vi "test Echo Frame.vi"(11 "Test Case In":refnum<class "Test PCANBasic.lvclass">) -> (0 "error out":errorcluster, 3 "Test Case Out":refnum<class "Test PCANBasic.lvclass">)   [LabVIEW 2020, in "Test PCANBasic.lvclass"]
uses:
  Test PCANBasic.lvclass
  C:/Program Files/National Instruments/LabVIEW 2026/vi.lib/Astemes/LUnit/Test Case.lvclass
  <vilib>/Astemes/LUnit/Test Case.lvclass/Test Case.ctl
  Test PCANBasic.lvclass/Test PCANBasic.ctl
  C:/Program Files/National Instruments/LabVIEW 2026/vi.lib/Astemes/LUnit/LUnit Runnable.lvclass
  D:/git/PCAN-Basic-LabVIEW/tests/Tests PCANBasic/Test PCANBasic.lvclass
  source/PCANBasic.lvlib
  Global PCAN Channel.vi
  Global PCAN Baudrate.vi
  <vilib>/Astemes/LUnit/Test Case.lvclass
panel:
  out "PCAN Message":T1 {"DATA"."7" format="%.0x"; "DATA"."6" format="%.0x"; "DATA"."5" format="%.0x"; "DATA"."4" format="%.0x"; "DATA"."3" format="%.0x"; "DATA"."2" format="%.0x"; "DATA"."1" format="%.0x"; "DATA"."0" format="%.0x"; "MSGTYPE"."Type" items=["STANDARD"=0, "RTR"=1, "ERRFRAME"=64, "STATUS"=128]}
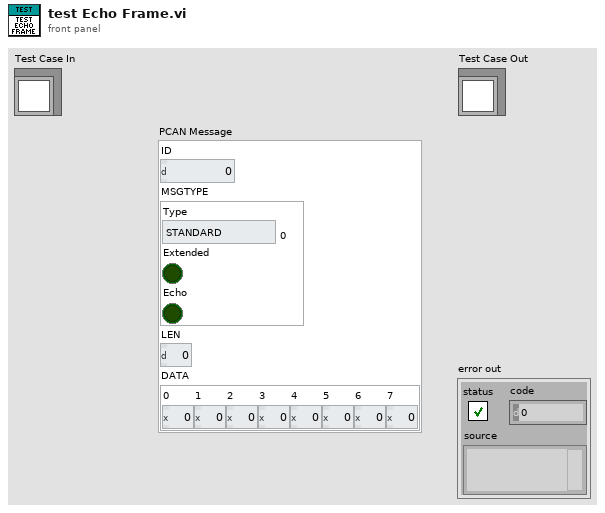
[diagram p1: front panel]
types:
  T1 = cluster{"ID":u32, "MSGTYPE":cluster{"Type":u8, "Extended":bool, "Echo":bool}, "LEN":u8, "DATA":cluster{"0":u8, "1":u8, "2":u8, "3":u8, "4":u8, "5":u8, "6":u8, "7":u8}}
  T2 = cluster{"0":u8, "1":u8, "2":u8, "3":u8, "4":u8, "5":u8, "6":u8, "7":u8}
  T3 = typedef "PCANBasic.lvlib/PCAN Baud.ctl" = u16
  T4 = typedef "PCANBasic.lvlib/TPCANHandle.ctl" = u16
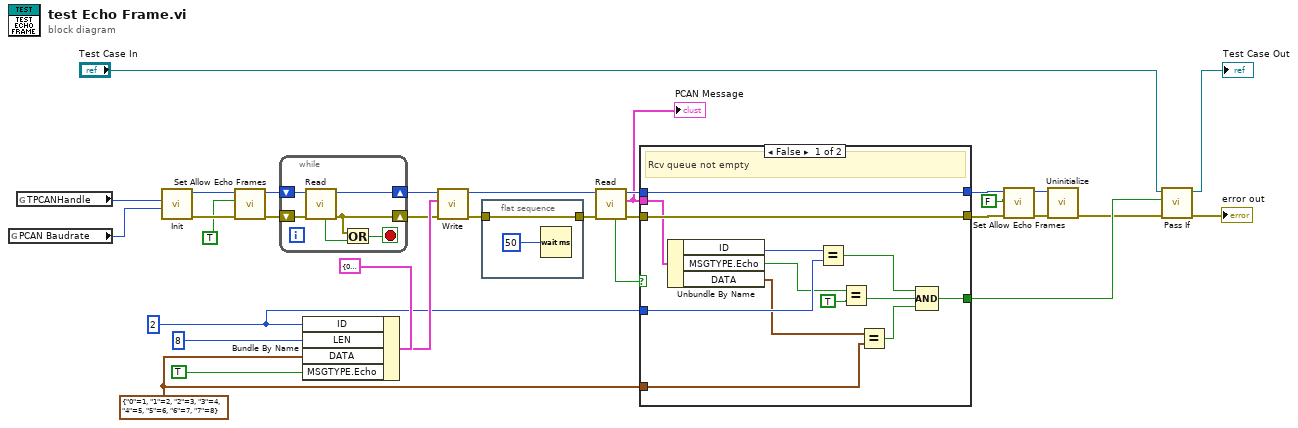
[diagram p0: block diagram]
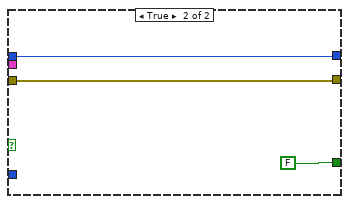
[diagram p2: hidden frame]
diagram:
  w16 = T2 {"0"=1, "1"=2, "2"=3, "3"=4, "4"=5, "5"=6, "6"=7, "7"=8} ("DATA")
  w17 = u32 2 ("ID")
  n1 = global read "Global PCAN Baudrate.vi" "PCAN Baudrate"() -> (w29:T3)
  n2 = global read "Global PCAN Channel.vi" "TPCANHandle"() -> (w28:T4)
  n3 = call "Init.vi"("Baudrate"=w29, "Channel"=w28) -> ("error out"=w27:errorcluster, "TPCANHandle out"=w12:T4)  [unwired: 7 in, 1 out]
  n4 = call "Set Allow Echo Frames.vi"("error in"=w27, "Enable"=TRUE, "TPCANHandle in"=w12) -> ("error out"=w13:errorcluster, "TPCANHandle out"=w10:T4)  [unwired: 6 in, 1 out]
  n5 = while {
    shift-right: [w34] -> w22
    shift-left: w13 -> [w38]
    shift-right: [w36] -> w21
    shift-left: w10 -> [w37]
    stop <- w33 stop-if-true
    n6 = call "Read.vi"("error in"=w38, "TPCANHandle in"=w37) -> ("error out"=w34:errorcluster, "TPCANHandle out"=w36:T4, "Receive Queue empty"=w35:bool)  [unwired: 4 in, 3 out]
    n7 = Or(x=w34, y=w35) -> (x .or. y?=w33:bool)
  }
  n8 = Bundle By Name(cluster=T1 {"ID"=0, "MSGTYPE"={"Type"=0, "Extended"=FALSE, "Echo"=FALSE}, "LEN"=0, "DATA"={"0"=0, "1"=0, "2"=0, "3"=0, "4"=0, "5"=0, "6"=0, "7"=0}} ("PCAN Message"), "ID"=w17, "LEN"=u8 8, "DATA"=w16, "MSGTYPE.Echo"=TRUE) -> (w24:T1)
  n9 = call "Write.vi"("error in"=w22, "PCAN Message"=w24, "TPCANHandle in"=w21) -> ("error out"=w7:errorcluster, "TPCANHandle out"=w19:T4)  [unwired: 6 in, 1 out]
  n10 = flat-sequence {
    tunnel: w7 -> [w40]
    tunnel: [w40] -> w6
    frame #0 {
      n11 = Wait (ms)(milliseconds to wait=u32 50) -> ()  [unwired: 1 out]
    }
  }
  n12 = call "Read.vi"("error in"=w6, "TPCANHandle in"=w19) -> ("error out"=w20:errorcluster, "PCAN Message"=w5:T1, "TPCANHandle out"=w18:T4, "Receive Queue empty"=w14:bool)  [unwired: 4 in, 2 out]
  "PCAN Message" <- w5
  n13 = case shown="False" w14 {
    tunnel: w20 -> [w43 w55]
    tunnel: w18 -> [w42 w54]
    tunnel: [w43 w55] -> w9
    tunnel: w5 -> [w41 _]
    tunnel: w17 -> [w53 _]
    tunnel: w16 -> [w48 _]
    tunnel: [w44 FALSE] -> w15
    tunnel: [w42 w54] -> w3
    frame False {
      # "Rcv queue not empty"
      n14 = Unbundle By Name(w41) -> ("ID"=w52:u32, "MSGTYPE.Echo"=w51:bool, "DATA"=w49:T2)
      n15 = Equal?(x=w52, y=w53) -> (x = y?=w47:bool)
      n16 = Equal?(x=w51, y=TRUE) -> (x = y?=w46:bool)
      n17 = Equal?(x=w49, y=w48) -> (x = y?=w45:bool)
      n18 = Compound Arithmetic op=AND(w47, w46, w45) -> (w44:bool)
    }
    frame True {
    }
  }
  n19 = call "Set Allow Echo Frames.vi"("error in"=w9, "Enable"=FALSE, "TPCANHandle in"=w3) -> ("error out"=w4:errorcluster, "TPCANHandle out"=w2:T4)  [unwired: 6 in, 1 out]
  n20 = call "Uninitialize.vi"("error in"=w4, "TPCANHandle in"=w2) -> ("error out"=w8:errorcluster)  [unwired: 8 in, 1 out]
  n21 = call <vilib>:"Pass If.vi"("error in (no error)"=w8, "Pass?"=w15, "LUnit Test Case In"="Test Case In") -> ("error out"=→"error out":errorcluster, "LUnit Test Case Out"=→"Test Case Out":refnum<class "Test PCANBasic.lvclass">)  [unwired: 7 in]
